vi "mCode.vi"(9 "Variable":cluster{"X":dbl, "Y":dbl, "Z":dbl}, 11 "mCode":T1) -> (2 "mCodeOut":string)   [LabVIEW 2017]
uses:
  controls/mCodeConfig.ctl
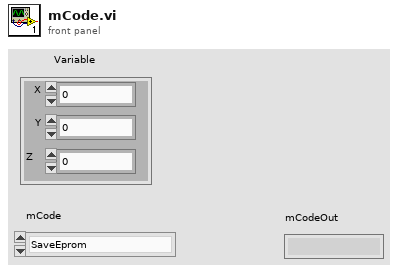
[diagram p1: front panel]
types:
  T1 = typedef "mCodeConfig.ctl" = enum16{"SaveEprom", "GetPosition", "SetAxisStepPerUnit", "EnableStep", "DisableStep", "PowerOn", "PowerOff", "EMGStop", "SerialPrint", "WaitforPinState", "SetMictoStep", "WaitFinishMove", "SetMaxFeedRate", "SetMaxACCEL", "SetStartACCEL", "SetSoleNoid", "SetFan1", "SetFan2", "SetFan3", "SetSpindle", "M5OffSpindle"}
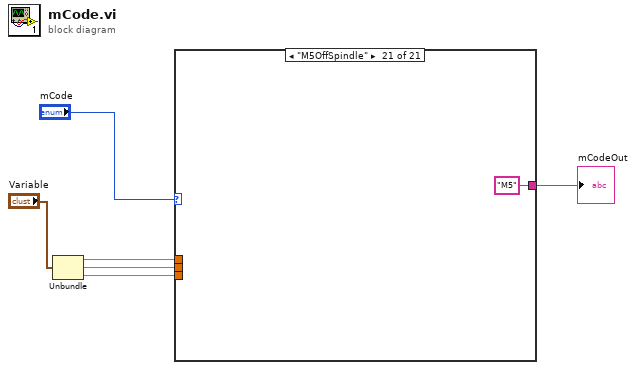
[diagram p0: block diagram]
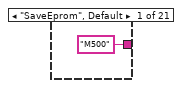
[diagram p2: hidden frame]
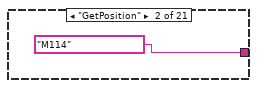
[diagram p3: hidden frame]
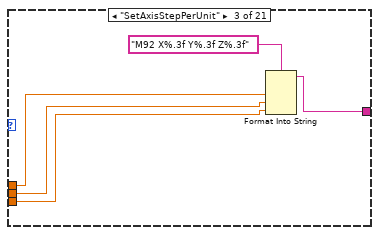
[diagram p4: hidden frame]
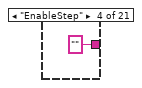
[diagram p5: hidden frame]
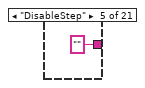
[diagram p6: hidden frame]
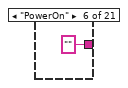
[diagram p7: hidden frame]
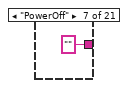
[diagram p8: hidden frame]
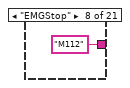
[diagram p9: hidden frame]
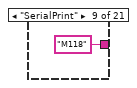
[diagram p10: hidden frame]
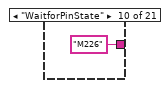
[diagram p11: hidden frame]
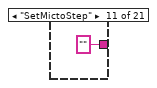
[diagram p12: hidden frame]
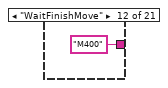
[diagram p13: hidden frame]
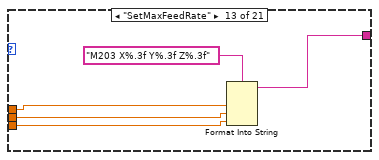
[diagram p14: hidden frame]
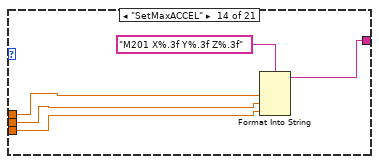
[diagram p15: hidden frame]
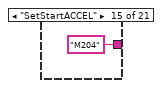
[diagram p16: hidden frame]
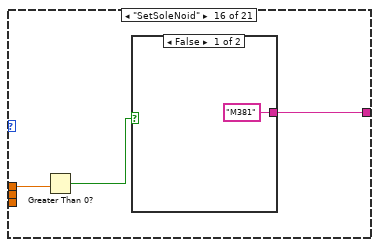
[diagram p17: hidden frame]
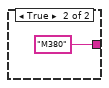
[diagram p18: hidden frame]
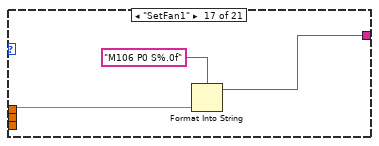
[diagram p19: hidden frame]
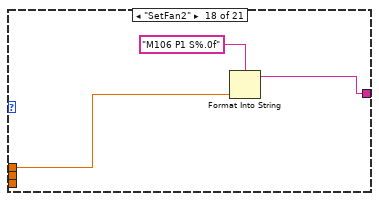
[diagram p20: hidden frame]
diagram:
  n1 = Unbundle("Variable") -> ("X"=w4:dbl, "Y"=w3:dbl, "Z"=w1:dbl)
  n2 = case shown="\"M5OffSpindle\"" "mCode" {
    tunnel: ["M500" "M114" w12 "" "" "" "" "M112" "M118" "M226" "" "M400" w23 w31 "M204" w34 w40 w43 w46 w49 "M5"] -> w5
    tunnel: w4 -> [_ _ w11 _ _ _ _ _ _ _ _ _ w26 w30 _ w36 w39 w42 w45 w48 _]
    tunnel: w3 -> [_ _ w10 _ _ _ _ _ _ _ _ _ w25 w29 _ _ _ _ _ _ _]
    tunnel: w1 -> [_ _ w9 _ _ _ _ _ _ _ _ _ w24 w28 _ _ _ _ _ _ _]
    frame "SaveEprom", Default {
    }
    frame "GetPosition" {
    }
    frame "SetAxisStepPerUnit" {
      n3 = Format Into String(format string="M92 X%.3f Y%.3f Z%.3f", w11, w10, w9) -> (resulting string=w12:string)  [unwired: 2 in, 1 out]
    }
    frame "EnableStep" {
    }
    frame "DisableStep" {
    }
    frame "PowerOn" {
    }
    frame "PowerOff" {
    }
    frame "EMGStop" {
    }
    frame "SerialPrint" {
    }
    frame "WaitforPinState" {
    }
    frame "SetMictoStep" {
    }
    frame "WaitFinishMove" {
    }
    frame "SetMaxFeedRate" {
      n4 = Format Into String(format string="M203 X%.3f Y%.3f Z%.3f", w26, w25, w24) -> (resulting string=w23:string)  [unwired: 2 in, 1 out]
    }
    frame "SetMaxACCEL" {
      n5 = Format Into String(format string="M201 X%.3f Y%.3f Z%.3f", w30, w29, w28) -> (resulting string=w31:string)  [unwired: 2 in, 1 out]
    }
    frame "SetStartACCEL" {
    }
    frame "SetSoleNoid" {
      n6 = Greater Than 0?(x=w36) -> (x > 0?=w35:bool)
      n7 = case shown="False" w35 {
        tunnel: ["M381" "M380"] -> w34
        frame False {
        }
        frame True {
        }
      }
    }
    frame "SetFan1" {
      n8 = Format Into String(format string="M106 P0 S%.0f", w39) -> (resulting string=w40:string)  [unwired: 2 in, 1 out]
    }
    frame "SetFan2" {
      n9 = Format Into String(format string="M106 P1 S%.0f", w42) -> (resulting string=w43:string)  [unwired: 2 in, 1 out]
    }
    frame "SetFan3" {
      n10 = Format Into String(format string="M106 P2 S%.0f", w45) -> (resulting string=w46:string)  [unwired: 2 in, 1 out]
    }
    frame "SetSpindle" {
      n11 = Format Into String(format string="M3 S%.0f", w48) -> (resulting string=w49:string)  [unwired: 2 in, 1 out]
    }
    frame "M5OffSpindle" {
    }
  }
  "mCodeOut" <- w5
